vi "acq.IncNum.vi"(7 "DVR in":T1, 8 "error in":errorcluster) -> (0 "error out":errorcluster)   [LabVIEW 2020]
uses:
  _controls/data.ref.ctl
  _controls/data.ctl
  _controls/state.ctl
  _controls/data.vars.ctl
  _controls/flip.ctl
  <vilib>/vision/Image Controls.llb/IMAQ Image.ctl
  camera/camera.lvclass
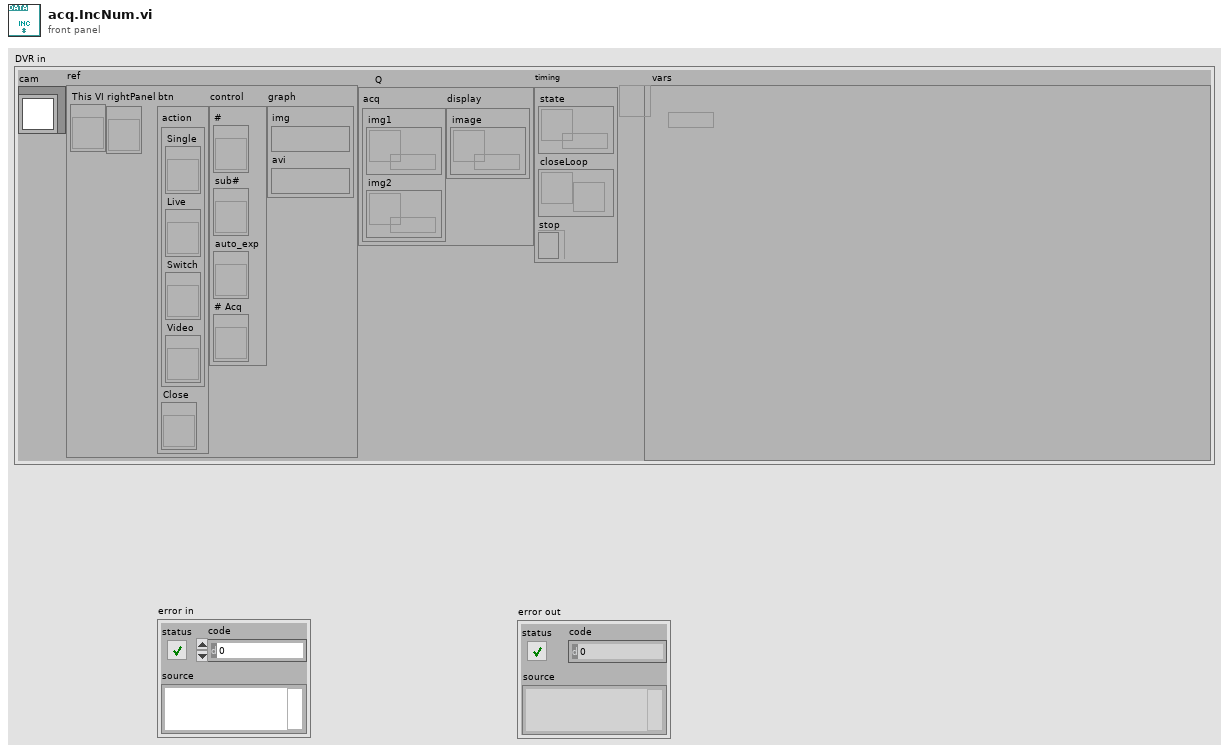
[diagram p1: front panel]
types:
  T1 = typedef "data.ctl" = cluster{"cam":refnum<class "camera.lvclass">, "ref":T2, "Q":cluster{"acq":cluster{"img1":refnum<queue>, "img2":refnum<queue>}, "display":cluster{"image":refnum<queue>}}, "timing":cluster{"state":refnum<queue>, "closeLoop":refnum<notifier>, "stop":refnum<k4>}, "vars":refnum<data-value>}
  T2 = typedef "data.ref.ctl" = cluster{"This VI":refnum<vi>, "rightPanel":refnum<vi>, "btn":cluster{"action":cluster{"Single":refnum<vi>, "Live":refnum<vi>, "Switch":refnum<vi>, "Video":refnum<vi>}, "Close":refnum<vi>}, "control":cluster{"#":refnum<vi>, "sub#":refnum<vi>, "auto_exp":refnum<vi>, "# Acq":refnum<vi>}, "graph":cluster{"img":T3, "avi":T3}}
  T3 = typedef "IMAQ Image.ctl" = refnum<image>
  T4 = typedef "data.vars.ctl" = cluster{"save":cluster{"base_folder":cluster{"Folder":path, "tif":bool, "jpg":bool}, "module":string, "#":u32, "sub#":u8, "save.op":enum16{"Full", "Light"}, "same?":bool, "Shift":enum16{"Single", "Leapfrog"}, "jpg?":bool, "flip":T5}, "acq":cluster{"# Acq":u16, "rotate":bool, "FPS":dbl}, "calib.manual":cluster{"BG":cluster{"Image":u16[][], "enabled?":bool}, "FF":cluster{"Image":u16[][], "enabled?":bool}}}
  T5 = typedef "flip.ctl" = cluster{"x":bool, "y":bool}
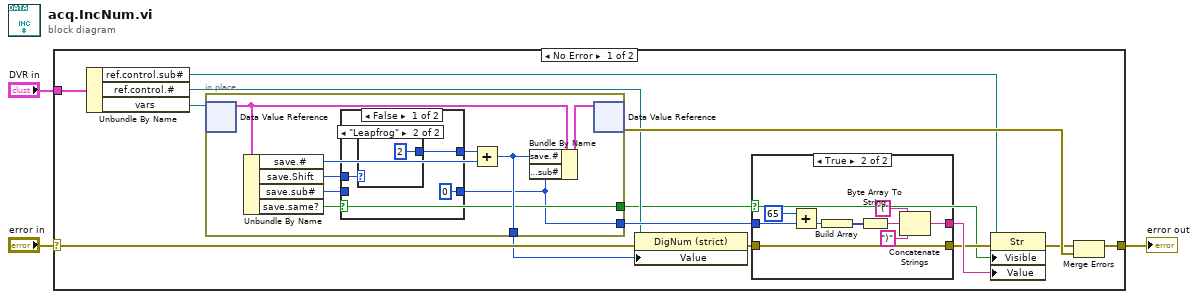
[diagram p0: block diagram]
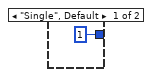
[diagram p3: hidden frame]
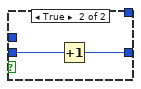
[diagram p4: hidden frame]
diagram:
  n1 = case shown="No Error" "error in" {
    selector: "error in" -> [w13 w44]
    tunnel: "DVR in" -> [w15 _]
    tunnel: [w14 w44] -> w2
    frame No Error {
      n2 = Unbundle By Name(w15) -> ("ref.control.sub#"=w5:refnum<vi>, "ref.control.#"=w8:refnum<vi>, "vars"=w16:refnum<data-value>)
      n3 = in-place {
        in-place-border: [w32] -> w12
        in-place-border: [w28] -> w10
        in-place-border: [w30] -> w4
        n4 = in-place-dvr #1(w16) -> (w35:T4)  [unwired: 1 out]
        n5 = Unbundle By Name(w35) -> ("save.#"=w34:u32, "save.Shift"=w33:enum16{"Single", "Leapfrog"}, "save.sub#"=w29:u8, "save.same?"=w30:bool)
        n6 = case shown="False" w30 {
          tunnel: w33 -> [w39 _]
          tunnel: [w38 _] -> w31
          tunnel: w29 -> [_ w43]
          tunnel: [u8 0 ("f") w42] -> w28
          frame False {
            n7 = case shown="\"Leapfrog\"" w39 {
              tunnel: [1 ("#") 2 ("#")] -> w38
              frame "Single", Default {
              }
              frame "Leapfrog" {
              }
            }
          }
          frame True {
            n8 = Increment(x=w43) -> (x+1=w42:u8)
          }
        }
        n9 = Add(x=w31, y=w34) -> (x+y=w32:u32)
        n10 = Bundle By Name(cluster=w35, "save.#"=w32, "save.sub#"=w28) -> (w36:T4)
        n11 = in-place-dvr #1(w36) -> (w17:errorcluster)  [unwired: 1 out]
      }
      n12 = property class="DigNum (strict)"(reference=w8, error in=w13, "Value"=w12) -> (error out=w7:errorcluster)  [unwired: 1 out]
      n13 = case shown="True" w4 {
        tunnel: w10 -> [_ w27]
        tunnel: [_ w24] -> w9
        tunnel: w7 -> [w18 w19]
        tunnel: [w18 w19] -> w6
        frame False {
        }
        frame True {
          n14 = Add(x=u8 65, y=w27) -> (x+y=w21:u8)
          n15 = Build Array(w21) -> (w26:u8[])
          n16 = Byte Array To String(unsigned byte array=w26) -> (string=w25:string)
          n17 = Concatenate Strings("(" ("string"), w25, ")" ("string")) -> (w24:string)
        }
      }
      n18 = property class="Str"(reference=w5, error in=w6, "Visible"=w4, "Value"=w9) -> (error out=w11:errorcluster)  [unwired: 1 out]
      n19 = Merge Errors(w11, w17) -> (w14:errorcluster)
    }
    frame Error {
    }
  }
  "error out" <- w2
